vi "Thermo Gas Conc Read Single Instr. (SubVI).vi"(0 "IP Address":string="192.168.1.201", 1 "Remore Port":u16=502, 5 "Quantity Register":u16=6, 7 "Units":string="ppb", 9 "MBAP Header":cluster{"Transaction ID":u16, "Unit ID":u8}={"Transaction ID"=0, "Unit ID"=42}, 11 "Error In":errorcluster) -> (4 "Data Out":T1(array[cluster]), 15 "error out":errorcluster)   [LabVIEW 2012]
uses:
  <vilib>/Utility/error.llb/DialogType.ctl
  Program Files/National Instruments/LabVIEW 2012/vi.lib/NI Modbus.llb/MB Ethernet Master Query Read Holding Registers (poly).vi
panel:
  in  "Starting Address":u16
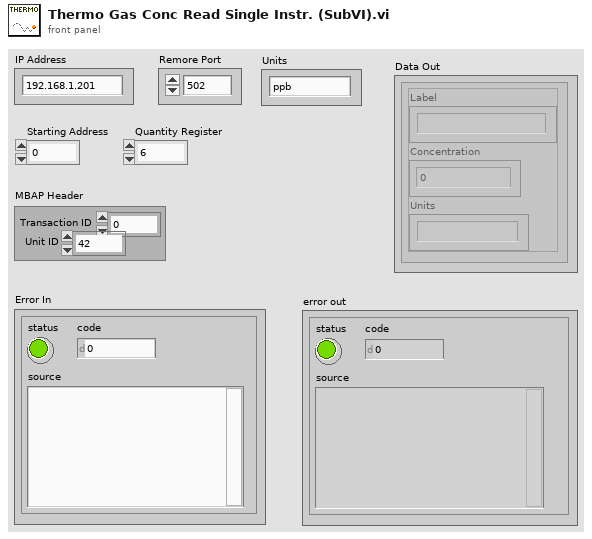
[diagram p1: front panel]
types:
  T1 = cluster{"Label":string, "Concentration":sgl, "Units":string}[]
  T2 = typedef "DialogType.ctl" = u16
  T3 = cluster{"Label":string, "Concentration":sgl, "Units":string}
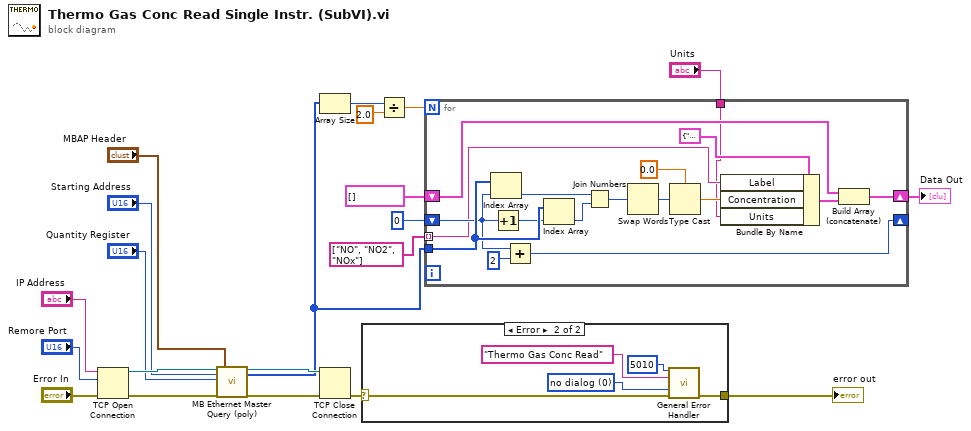
[diagram p0: block diagram]
diagram:
  n1 = TCP Open Connection(address="IP Address", remote port or service name="Remore Port", error in (no error)="Error In") -> (connection ID=w19:refnum<k5>, error out=w18:errorcluster)  [unwired: 2 in]
  n2 = call-poly "MB Ethernet Master Query (poly).vi"("TCP Connection Refnum in"=w19, "Starting Address"="Starting Address", "Quantity"="Quantity Register", "error in"=w18, "MBAP Header"="MBAP Header") -> ("TCP Connection Refnum (dup)"=w21:refnum<k5>, "Holding Registers"=w9:u16[], "error out"=w20:errorcluster)  [unwired: 11 in, 1 out]
  n3 = Array Size(array=w9) -> (size(s)=w14:i32)
  n4 = TCP Close Connection(connection ID=w21, error in (no error)=w20) -> (error out=w3:errorcluster)  [unwired: 1 in, 1 out]
  n5 = case shown="Error" w3 {
    selector: w3 -> [w22 w24]
    tunnel: [w22 w23] -> w2
    frame No Error {
    }
    frame Error {
      w25 = T2 0 items=["no dialog", "OK message", "continue or stop message", "OK message + warnings", "continue/stop + warnings"] ("type of dialog (OK msg:1)")
      n6 = call <vilib>:"General Error Handler.vi"("[error code] (0)"=5010, "[error source] (\" \")"="Thermo Gas Conc Read" ("[error source] (\" \")"), "type of dialog (OK msg:1)"=w25, "error in (no error)"=w24) -> ("error out"=w23:errorcluster)  [unwired: 7 in, 4 out]
    }
  }
  "error out" <- w2
  n7 = Divide(x=w14, y=2.0) -> (x/y=w13:dbl)
  n8 = for {
    N: w13 -> [_]
    tunnel: w9 -> [w44]
    shift-right: [w31] -> w10
    shift-left: T1 [] -> [w30]
    shift-right: [w37] -> _
    shift-left: 0 -> [w35]
    tunnel: string[] ["NO", "NO2", "NOx"] -> [w29] mode=indexing
    tunnel: "Units" -> [w28]
    n9 = Index Array(array=w44, index=w35) -> (element=w41:u16)
    n10 = Increment(x=w35) -> (x+1=w34:i32)
    n11 = Add(x=w35, y=2) -> (x+y=w37:i32)
    n12 = Index Array(array=w44, index=w34) -> (element=w40:u16)
    n13 = Join Numbers(hi=w41, lo=w40) -> ((hi.lo)=w42:u32)
    n14 = Swap Words(1:w42) -> (0:w39:u32)
    n15 = Type Cast(type=sgl 0.0, x=w39) -> (*(type *) &x=w38:sgl)
    n16 = Bundle By Name(cluster=T3 {"Label"="", "Concentration"=0.0, "Units"=""}, "Label"=w29, "Concentration"=w38, "Units"=w28) -> (w33:T3)
    n17 = Build Array (concatenate)(w30, w33) -> (w31:T1)
  }
  "Data Out" <- w10
